vi "Initialize Camera.vi"() -> (1 "Cluster":cluster{"value":i32, "value":i32, "index":i32}, 2 "Array":cluster{string[]}[](array[cluster]), 3 "File Refnum":T1)   [LabVIEW 2015]
uses:
  <vilib>/Utility/config.llb/Config Data RefNum.ctl
  <vilib>/Utility/config.llb/Read Key (String).vi
  <vilib>/Utility/config.llb/Read Key (I32).vi
  <vilib>/Utility/config.llb/NI_LVConfig.lvlib
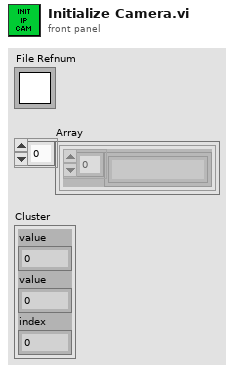
[diagram p1: front panel]
types:
  T1 = typedef "NI_LVConfig.lvlib/Config Data RefNum.ctl" = refnum<k1>
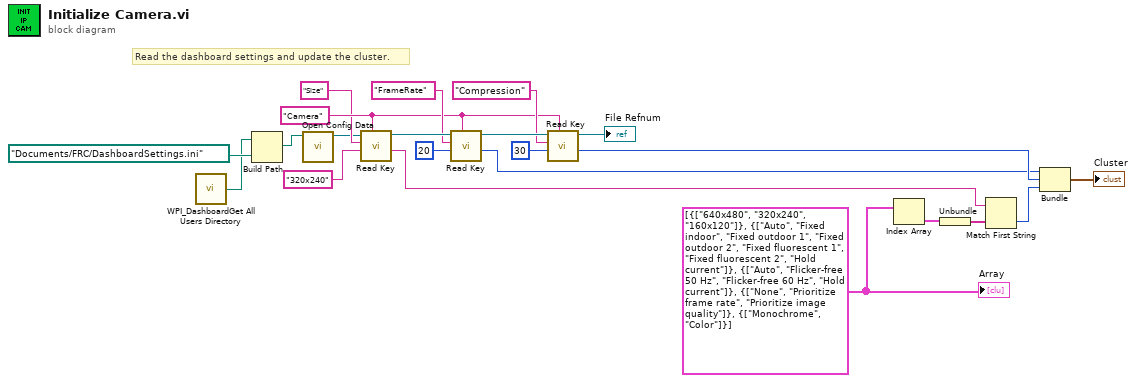
[diagram p0: block diagram]
diagram:
  w6 = "Camera"
  w14 = cluster{string[]}[] [{["640x480", "320x240", "160x120"]}, {["Auto", "Fixed indoor", "Fixed outdoor 1", "Fixed outdoor 2", "Fixed fluorescent 1", "Fixed fluorescent 2", "Hold current"]}, {["Auto", "Flicker-free 50 Hz", "Flicker-free 60 Hz", "Hold current"]}, {["None", "Prioritize frame rate", "Prioritize image quality"]}, {["Monochrome", "Color"]}]
  # "Read the dashboard settings and update the cluster."
  n1 = call <vilib>:"WPI_DashboardGet All Users Directory.vi"() -> ("All User Path"=w1:path)
  n2 = Build Path(base path=w1, name or relative path=path "Documents/FRC/DashboardSettings.ini") -> (appended path=w2:path)
  n3 = call <vilib>:"Open Config Data.vi"("configuration file path"=w2) -> ("refnum"=w3:T1)  [unwired: 8 in, 2 out]
  n4 = call-poly <vilib>:"Read Key.vi"("section"=w6, "default value"="320x240", "key"="Size", "refnum"=w3) -> ("value"=w16:string, "refnum out"=w19:T1)  [unwired: 2 in, 4 out]
  n5 = call-poly <vilib>:"Read Key.vi"("section"=w6, "default value"=20, "key"="FrameRate", "refnum"=w19) -> ("value"=w11:i32, "refnum out"=w20:T1)  [unwired: 1 in, 5 out]
  n6 = call-poly <vilib>:"Read Key.vi"("section"=w6, "default value"=30, "key"="Compression", "refnum"=w20) -> ("value"=w12:i32, "refnum out"=→"File Refnum":T1)  [unwired: 1 in, 5 out]
  n7 = Index Array(array=w14) -> (element=w13:cluster{string[]})  [unwired: 1 in]
  n8 = Unbundle(w13) -> (w15:string[])
  n9 = Match First String(2:w15, 3:w16) -> (0:w17:i32)  [unwired: 1 out]
  n10 = Bundle("value"=w11, "value"=w12, "index"=w17) -> (→"Cluster":cluster{"value":i32, "value":i32, "index":i32})  [unwired: 1 out]
  "Array" <- w14
